vi "Save Document.vi"(8 "error in (no error)":errorcluster, 11 "Document in":refnum<class "Document.lvclass">) -> (0 "error out":errorcluster, 3 "Document out":refnum<class "Document.lvclass">)   [LabVIEW 2017, in "LabVIEW NPOI.lvlib" / "Document.lvclass"]
doc: "Saves the <b>Document</b> to the <b>File Path</b> location given in the create or open method."
uses:
  Document.lvclass
  Document.lvclass/Document.ctl
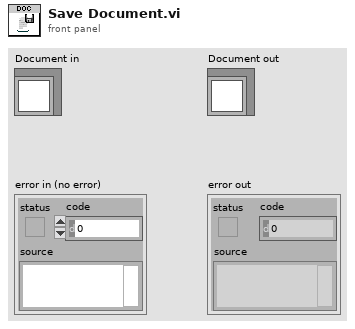
[diagram p1: front panel]
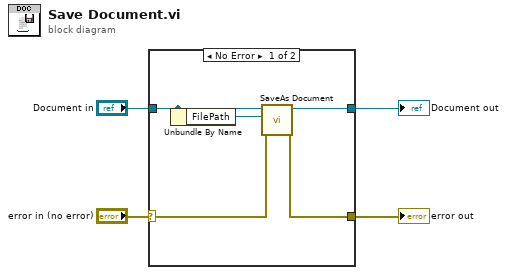
[diagram p0: block diagram]
diagram:
  n1 = case shown="No Error" "error in (no error)" {
    selector: "error in (no error)" -> [w8 w11]
    tunnel: [w7 w11] -> w3
    tunnel: [w9 w10] -> w1
    tunnel: "Document in" -> [w6 w10]
    frame No Error {
      n2 = Unbundle By Name(w6) -> ("FilePath"=w5:path)
      n3 = call "SaveAs Document.vi"("error in (no error)"=w8, "File Path"=w5, "Document in"=w6) -> ("error out"=w7:errorcluster, "Document out"=w9:refnum<class "Document.lvclass">)  [unwired: 7 in]
    }
    frame Error {
    }
  }
  "error out" <- w3
  "Document out" <- w1
